vi "1D_to_2D_sub.vi"(1 "1D":dbl[](array[numeric])) -> (0 "2D(28_28)":dbl[][](array[numeric]))   [LabVIEW 2021]
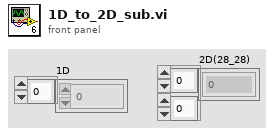
[diagram p1: front panel]
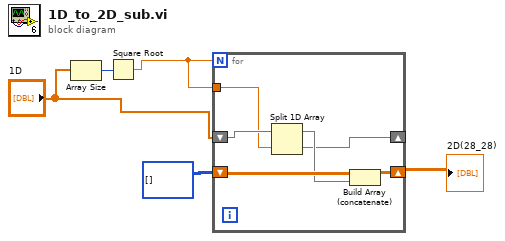
[diagram p0: block diagram]
diagram:
  n1 = Array Size(array="1D") -> (size(s)=w2:i32)
  n2 = Square Root(x=w2) -> (sqrt(x)=w1:dbl)
  n3 = for {
    N: w1 -> [_]
    shift-right: [w11] -> w4
    shift-left: i32[][] [] -> [w10]
    shift-right: [w8] -> _
    shift-left: "1D" -> [w7]
    tunnel: w1 -> [w6]
    n4 = Split 1D Array(array=w7, index=w6) -> (first subarray=w9:dbl[], second subarray=w8:dbl[])
    n5 = Build Array (concatenate)(w10, w9) -> (w11:dbl[][])
  }
  "2D(28_28)" <- w4
